vi "FPGA Latch.vi"(11 "Input":bool) -> (3 "Latch?":bool)   [LabVIEW 2015, in "FPGA_shared.lvlib"]
uses:
  FPGA_shared.lvlib
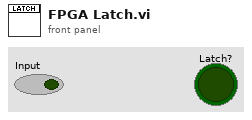
[diagram p1: front panel]
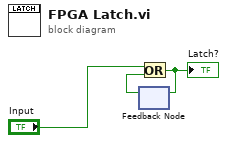
[diagram p0: block diagram]
diagram:
  n1 = feedback #1() -> (w1:bool)  [unwired: 1 in]
  n2 = Or(x="Input", y=w1) -> (x .or. y?=w3:bool)
  "Latch?" <- w3
  n3 = feedback-in #1(w3) -> ()
